vi "Change Month.vi"(8 "Display State In":cluster{"Month":i32, "Day":i32, "Year":i32}={"Month"=1, "Day"=1, "Year"=2022}, 11 "Change":enum16{"Next", "Last"}(ring)) -> (0 "Display State Out":cluster{"Month":i32, "Day":i32, "Year":i32}={"Month"=1, "Day"=1, "Year"=2022})   [LabVIEW 2019, in "Custom Calendar.xctl"]
uses:
  Custom Calendar.xctl
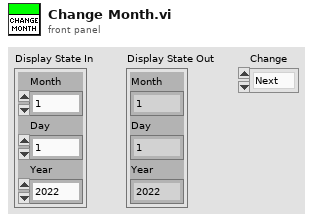
[diagram p1: front panel]
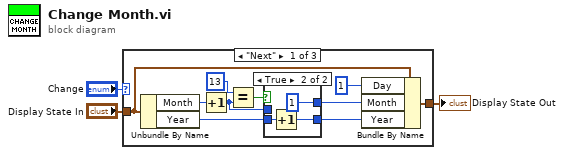
[diagram p0: block diagram]
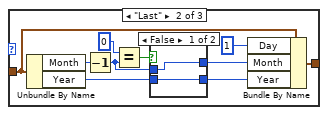
[diagram p3: hidden frame]
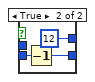
[diagram p4: hidden frame]
diagram:
  n1 = case shown="\"Next\"" "Change" {
    tunnel: "Display State In" -> [w10 w21 w34]
    tunnel: [w6 w20 w34] -> w1
    frame "Next" {
      n2 = Unbundle By Name(w10) -> ("Month"=w13:i32, "Year"=w8:i32)
      n3 = Increment(x=w13) -> (x+1=w5:i32)
      n4 = Equal?(x=13, y=w5) -> (x = y?=w11:bool)
      n5 = case shown="True" w11 {
        tunnel: [w15 1 ("x")] -> w9
        tunnel: w8 -> [w14 w17]
        tunnel: [w14 w16] -> w7
        tunnel: w5 -> [w15 _]
        frame False {
        }
        frame True {
          n6 = Increment(x=w17) -> (x+1=w16:i32)
        }
      }
      n7 = Bundle By Name(cluster=w10, "Day"=1, "Month"=w9, "Year"=w7) -> (w6:cluster{"Month":i32, "Day":i32, "Year":i32})
    }
    frame "Last" {
      n8 = Unbundle By Name(w21) -> ("Month"=w28:i32, "Year"=w24:i32)
      n9 = Decrement(x=w28) -> (x-1=w22:i32)
      n10 = Equal?(x=0, y=w22) -> (x = y?=w26:bool)
      n11 = case shown="False" w26 {
        tunnel: [w30 12 ("x")] -> w25
        tunnel: w24 -> [w29 w32]
        tunnel: [w29 w31] -> w23
        tunnel: w22 -> [w30 _]
        frame False {
        }
        frame True {
          n12 = Decrement(x=w32) -> (x-1=w31:i32)
        }
      }
      n13 = Bundle By Name(cluster=w21, "Day"=1, "Month"=w25, "Year"=w23) -> (w20:cluster{"Month":i32, "Day":i32, "Year":i32})
    }
    frame Default {
    }
  }
  "Display State Out" <- w1
